vi "Initialize AI Task.vi"(8 "error in (no error)":errorcluster, 11 "BNT_ULx-MCSV-TC in":refnum<class "BNT_ULx-MCSV-TC.lvclass">) -> (0 "error out":errorcluster, 3 "AI ULx Task":refnum<k24>)   [LabVIEW 2020, in "BNT_ULx.lvlib" / "BNT_ULx-MCSV-TC.lvclass"]
doc: "Initialize DAQmx Analog Input task.\n\n<b>Default Implementation:</b> Analog Input Voltage\n\nThis dynamic dispatch VI can be overritten by derived classes to implement other analog input tasks."
uses:
  BNT_ULx-MCSV-TC.lvclass
  C:/User/Brand/LVP/CSPP/CSPP-Template/Packages/CSPP_Core/Actors/CSPP_BaseActor/CSPP_BaseActor.lvclass
  C:/User/Brand/LVP/CSPP/CSPP-Template/Packages/BNT_ULx/BNT_ULx-MCSV/BNT_ULx-MCSV/BNT_ULx-MCSV.lvclass
  C:/Program Files (x86)/National Instruments/LabVIEW 2020/vi.lib/ULx/ULx_LV.dll
  Program Files (x86)/National Instruments/LabVIEW 2020/vi.lib/ULx/ULx_LV.dll
  CSPP_Core/Actors/CSPP_BaseActor/CSPP_BaseActor.lvclass/CSPP_BaseActor.ctl
  BNT_ULx-MCSV-TC.lvclass/BNT_ULx-MCSV-TC.ctl
  BNT_ULx-MCSV/BNT_ULx-MCSV.lvclass/BNT_ULx-MCSV.ctl
  CSPP_Core/Actors/CSPP_BaseActor/Read Object Name.vi
  Read CJC Channel.vi
  Read CJC Source.vi
  BNT_ULx-MCSV/Read AI Min.vi
  BNT_ULx-MCSV/Read AI Max.vi
  BNT_ULx-MCSV/Read AI ULx Physical Channels.vi
  Read Thermocouple Type.vi
  Read CJC Value.vi
  <vilib>/ULx/Create Channel.llb/ULx Create Channel (AI-Temperature).vi
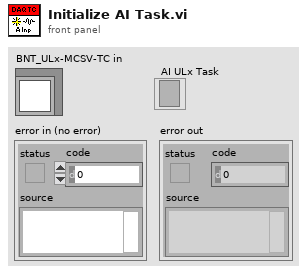
[diagram p1: front panel]
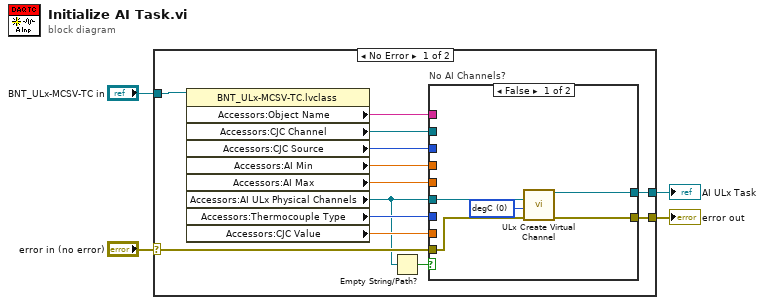
[diagram p0: block diagram]
diagram:
  n1 = case shown="No Error" "error in (no error)" {
    selector: "error in (no error)" -> [w17 w24]
    tunnel: [w9 w24] -> w3
    tunnel: "BNT_ULx-MCSV-TC in" -> [w16 _]
    tunnel: [w5 _] -> w1
    frame No Error {
      n2 = property class="BNT_ULx-MCSV-TC.lvclass"(reference=w16) -> ("Accessors:Object Name"=w8:string, "Accessors:CJC Channel"=w12:refnum<k21>, "Accessors:CJC Source"=w13:i32, "Accessors:AI Min"=w14:dbl, "Accessors:AI Max"=w15:dbl, "Accessors:AI ULx Physical Channels"=w7:refnum<k21>, "Accessors:Thermocouple Type"=w11:i32, "Accessors:CJC Value"=w10:dbl)  [unwired: 1 in, 2 out]
      n3 = Empty String/Path?(string/path=w7) -> (empty?=w6:bool)
      n4 = case "No AI Channels?" shown="False" w6 {
        tunnel: w17 -> [w20 w23]
        tunnel: w7 -> [w22 _]
        tunnel: w15 -> [_ _]
        tunnel: w14 -> [_ _]
        tunnel: w13 -> [_ _]
        tunnel: w12 -> [_ _]
        tunnel: w11 -> [_ _]
        tunnel: w10 -> [_ _]
        tunnel: [w19 w23] -> w9
        tunnel: w8 -> [_ _]
        tunnel: [w21 _] -> w5
        frame False {
          w18 = 0 items=["degC", "degF", "kelvin", "raw"] ("units")
          n5 = call-poly <vilib>:"ULx Create Virtual Channel.vi"("physical channels"=w22, "units"=w18, "error in"=w20) -> ("task out"=w21:refnum<k24>, "error out"=w19:errorcluster)  [unwired: 11 in]
        }
        frame True {
        }
      }
    }
    frame Error {
    }
  }
  "error out" <- w3
  "AI ULx Task" <- w1
